vi "draw_box.vi"(0 "Image in":refnum<class "Image.lvclass">, 1 "group":string, 5 "Box.lvclass":refnum<class "Box.lvclass">, 9 "depth":dbl[unit], 11 "error in (no error)":errorcluster, 12 "colour":u32(colorbox)=16711680, 13 "drawing mode (Frame)":u32(ring) items=["Frame", "Fill", "Highlight"]) -> (4 "Image out":refnum<class "Image.lvclass">, 15 "error out":errorcluster)   [LabVIEW 2010, in "Image.lvclass"]
uses:
  Image.lvclass
  Box/Box/Box.lvclass
  ErrorController/ErrorController/class_data.vi
  SpaceVector/SpaceVector/SpaceVector.lvclass
  ErrorController/ErrorController/ErrorController.lvclass
panel:
  # "This method draws the section of a 3D box with an image plane as an overlay."
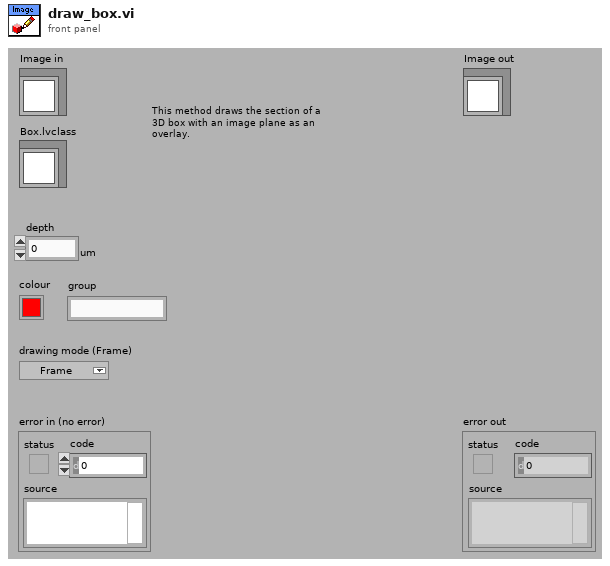
[diagram p1: front panel]
types:
  T1 = cluster{"[0]":i32, "[1]":i32, "[2]":i32, "[3]":i32}
  T2 = typedef "IMAQ Image.ctl" = refnum<image>
  T3 = typedef "space_vector_array.ctl" = dbl[unit][]
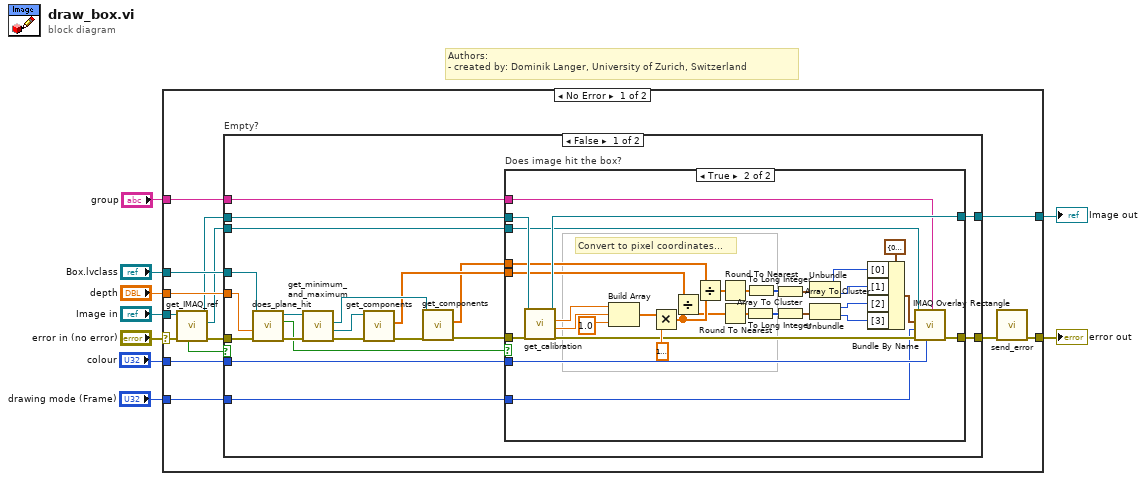
[diagram p0: block diagram]
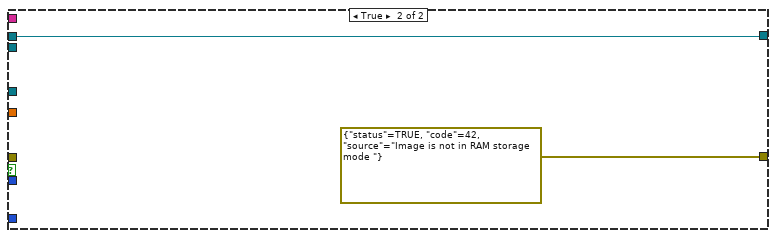
[diagram p3: hidden frame]
diagram:
  # "Authors: \n- created by: Dominik Langer, University of Zurich, Switzerland"
  n1 = case shown="No Error" "error in (no error)" {
    selector: "error in (no error)" -> [w20 w80]
    tunnel: [w11 w80] -> w8
    tunnel: [w15 w79] -> w6
    tunnel: "Image in" -> [w22 w79]
    tunnel: "Box.lvclass" -> [w23 _]
    tunnel: "depth" -> [w21 _]
    tunnel: "colour" -> [w14 _]
    tunnel: "group" -> [w13 _]
    tunnel: "drawing mode (Frame)" -> [w12 _]
    frame No Error {
      n2 = call-dynamic "get_IMAQ_ref.vi"("error in (no error)"=w20, "Image.lvclass in"=w22) -> ("error out"=w19:errorcluster, "Image"=w17:T2, "Image.lvclass out"=w16:refnum<class "Image.lvclass">, "empty?"=w18:bool)  [unwired: 5 in, 1 out]
      n3 = case "Empty?" shown="False" w18 {
        tunnel: w23 -> [w27 _]
        tunnel: w21 -> [w31 _]
        tunnel: w19 -> [w30 _]
        tunnel: [w38 errorcluster {"status"=TRUE, "code"=42, "source"="Image is not in RAM storage mode "} ("error out")] -> w10
        tunnel: w17 -> [w25 _]
        tunnel: w16 -> [w37 w77]
        tunnel: [w36 w77] -> w15
        tunnel: w14 -> [w33 _]
        tunnel: w13 -> [w32 _]
        tunnel: w12 -> [w24 _]
        frame False {
          n4 = call "does_plane_hit.vi"("error in (no error)"=w30, "depth"=w31, "Box in"=w27) -> ("error out"=w29:errorcluster, "is inside?"=w28:bool, "Box out"=w26:refnum<class "Box.lvclass">)  [unwired: 6 in]
          n5 = call "get_minimum_and_maximum.vi"("error in (no error)"=w29, "Box in"=w26) -> ("error out"=w42:errorcluster, "maximum"=w41:refnum<class "SpaceVector.lvclass">, "minimum"=w40:refnum<class "SpaceVector.lvclass">)  [unwired: 6 in, 1 out]
          n6 = call "get_components.vi"("error in (no error)"=w42, "SpaceVector in"=w41) -> ("error out"=w43:errorcluster, "x/y/z"=w35:T3)  [unwired: 4 in, 4 out]
          n7 = call "get_components.vi"("error in (no error)"=w43, "SpaceVector in"=w40) -> ("error out"=w39:errorcluster, "x/y/z"=w34:T3)  [unwired: 4 in, 4 out]
          n8 = case "Does image hit the box?" shown="True" w28 {
            tunnel: w39 -> [w45 w76]
            tunnel: [w45 w63] -> w38
            tunnel: w25 -> [_ w48]
            tunnel: w37 -> [w44 w75]
            tunnel: [w44 w74] -> w36
            tunnel: w35 -> [_ w70]
            tunnel: w34 -> [_ w69]
            tunnel: w33 -> [_ w62]
            tunnel: w32 -> [_ w61]
            tunnel: w24 -> [_ w46]
            frame False {
            }
            frame True {
              # "Convert to pixel coordinates..."
              n9 = call "get_calibration.vi"("error in (no error)"=w76, "Image.lvclass in"=w75) -> ("error out"=w47:errorcluster, "y"=w72:dbl, "x"=w73:dbl, "Image.lvclass out"=w74:refnum<class "Image.lvclass">)  [unwired: 4 in, 2 out]
              n10 = Build Array(w73, w72, 1.0 ("element")) -> (w68:dbl[])
              n11 = Multiply(x=w68, y=dbl[unit] 1e-06 ("element")) -> (x*y=w66:dbl[unit][])
              n12 = Divide(x=w70, y=w66) -> (x/y=w59:dbl[])
              n13 = Divide(x=w69, y=w66) -> (x/y=w60:dbl[])
              n14 = Round To Nearest(number=w60) -> (nearest integer value=w65:dbl[])
              n15 = Round To Nearest(number=w59) -> (nearest integer value=w64:dbl[])
              n16 = To Long Integer(number=w64) -> (32bit integer=w55:i32[])
              n17 = To Long Integer(number=w65) -> (32bit integer=w56:i32[])
              n18 = Array To Cluster(array=w56) -> (cluster=w54:cluster{"[0]":i32, "[1]":i32})
              n19 = Array To Cluster(array=w55) -> (cluster=w53:cluster{"[0]":i32, "[1]":i32})
              n20 = Unbundle(w54) -> ("[0]"=w52:i32, "[1]"=w51:i32)
              n21 = Unbundle(w53) -> ("[0]"=w50:i32, "[1]"=w49:i32)
              n22 = Bundle By Name(cluster=T1 {"[0]"=0, "[1]"=0, "[2]"=0, "[3]"=0}, "[0]"=w52, "[1]"=w51, "[2]"=w50, "[3]"=w49) -> (w57:T1)
              n23 = call "IMAQ Overlay Rectangle"("Color"=w62, "Group"=w61, "error in (no error)"=w47, "Drawing Mode (Frame)"=w46, "Rectangle"=w57, "Image"=w48) -> ("error out"=w63:errorcluster)  [unwired: 4 in, 1 out]
            }
          }
        }
        frame True {
        }
      }
      n24 = call "send_error.vi"("error in (no error)"=w10) -> ("error out"=w11:errorcluster)  [unwired: 10 in]
    }
    frame Error {
    }
  }
  "error out" <- w8
  "Image out" <- w6
